vi "Add the selected MANU test step for AUTO.vi"(8 "error in":errorcluster, 10 "Selected the MANU test Step to ADD":u8=1 min=1 max=100, 11 "VISA resource name":refnum<visa-resource-name>) -> (0 "error out":errorcluster, 3 "VISA resource name out":refnum<visa-resource-name>)   [LabVIEW 2011, in "GPT-9000.lvlib"]
uses:
  <instrlib>/GPT-9000/GPT-9000.lvlib
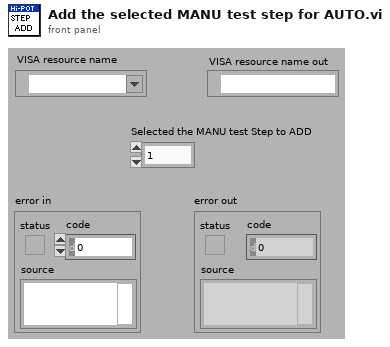
[diagram p1: front panel]
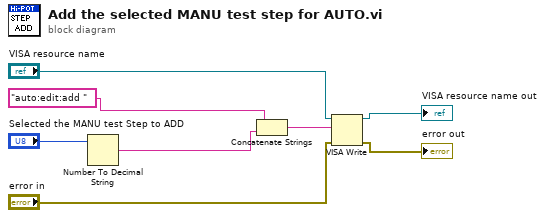
[diagram p0: block diagram]
diagram:
  n1 = Number To Decimal String(number="Selected the MANU test Step to ADD") -> (decimal integer string=w6:string)  [unwired: 1 in]
  n2 = Concatenate Strings("auto:edit:add ", w6) -> (w3:string)
  n3 = VISA Write(VISA resource name="VISA resource name", write buffer=w3, error in (no error)="error in") -> (VISA resource name out=→"VISA resource name out":refnum<visa-resource-name>, error out=→"error out":errorcluster)  [unwired: 1 out]
